vi "Mouse Up.vi"(8 "error in (no error)":errorcluster, 10 "Point":T1, 11 "Ellipse in":refnum<class "Ellipse.lvclass">) -> (0 "error out":errorcluster, 3 "Ellipse out":refnum<class "Ellipse.lvclass">)   [LabVIEW 2020, in "Ellipse.lvclass"]
doc: "A method for specifying how an ellipse reacts on a mouse up event"
uses:
  Ellipse.lvclass
  D:/Git/Labview-Libraries/Tools/Drawing Tool Folder/Graphics Object/Graphics Object.lvclass
  <vilib>/Utility/miscctls.llb/LVPoint32TypeDef.ctl
  Ellipse.lvclass/Ellipse.ctl
  Graphics Object/Graphics Object.lvclass
panel:
  # "expressionflow.com"
  # "Copyright (c) 2008 Tomi Maila. All rights reserved."
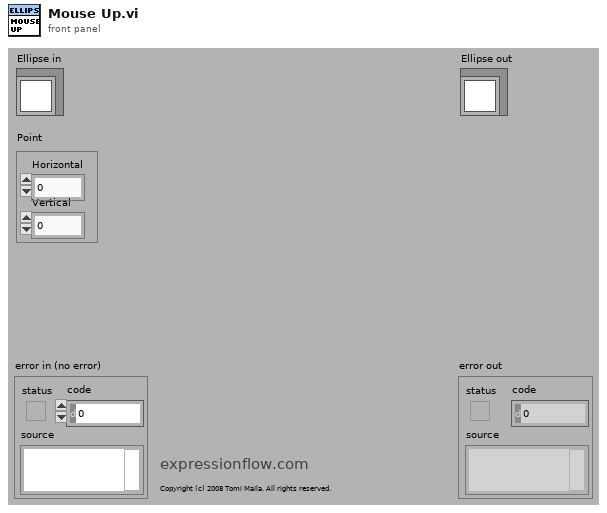
[diagram p1: front panel]
types:
  T1 = typedef "LVPoint32TypeDef.ctl" = cluster{"Horizontal":i32, "Vertical":i32}
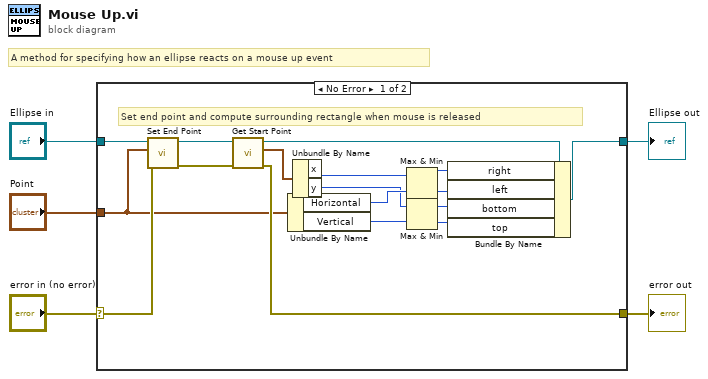
[diagram p0: block diagram]
diagram:
  # "A method for specifying how an ellipse reacts on a mouse up event"
  n1 = case shown="No Error" "error in (no error)" {
    selector: "error in (no error)" -> [w16 w23]
    tunnel: [w12 w23] -> w4
    tunnel: [w22 w24] -> w2
    tunnel: "Ellipse in" -> [w17 w24]
    tunnel: "Point" -> [w10 _]
    frame No Error {
      # "Set end point and compute surrounding rectangle when mouse is released"
      n2 = call "Set End Point.vi"("error in (no error)"=w16, "end point (0,0)"=w10, "Graphics Object.lvclass in"=w17) -> ("error out"=w13:errorcluster, "Graphics Object.lvclass out"=w15:refnum<class "Ellipse.lvclass">)  [unwired: 7 in]
      n3 = call "Get Start Point.vi"("error in (no error)"=w13, "Graphics Object.lvclass in"=w15) -> ("error out"=w12:errorcluster, "start point"=w11:cluster{"x":i16, "y":i16}, "Graphics Object.lvclass out"=w14:refnum<class "Ellipse.lvclass">)  [unwired: 7 in]
      n4 = Unbundle By Name(w10) -> ("Horizontal"=w9:i32, "Vertical"=w6:i32)
      n5 = Unbundle By Name(w11) -> ("x"=w8:i16, "y"=w7:i16)
      n6 = Max & Min(x=w8, y=w9) -> (max(x,y)=w21:i32, min(x,y)=w20:i32)
      n7 = Max & Min(x=w7, y=w6) -> (max(x,y)=w19:i32, min(x,y)=w18:i32)
      n8 = Bundle By Name(cluster=w14, "right"=w21, "left"=w20, "bottom"=w19, "top"=w18) -> (w22:refnum<class "Ellipse.lvclass">)
    }
    frame Error {
    }
  }
  "error out" <- w4
  "Ellipse out" <- w2
